vi "DEMO Lock.vi"(1 "Input":bool) -> (0 "Output":bool)   [LabVIEW 2011]
uses:
  Robot Global Data.vi
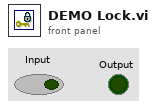
[diagram p1: front panel]
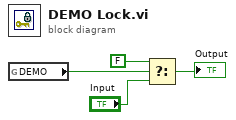
[diagram p0: block diagram]
diagram:
  n1 = global read "Robot Global Data.vi" "DEMO"() -> (w4:bool)
  n2 = Select(t=FALSE, s=w4, f="Input") -> (s? t:f=→"Output":bool)
